vi "SetBuildVersionCaller.vi"(11 "Command line arguments \nfor the VI":string[](array[string])) -> (2 "Output or error information to include in \nthe CLI for LabVIEW console or log file.":string, 3 "CLI for LabVIEW exit code that the VI returns":i32)   [LabVIEW 2020]
doc: "Calls SetBuildVersion.vi to set the version of the build specification."
uses:
  <vilib>/AppBuilder/AB_API_Simple/Build Specification Version.ctl
  <vilib>/AppBuilder/AB_API_Simple/NI_App_Builder_API.lvlib
  <vilib>/AdvancedString/1D String Array to Delimited String (string).vi
  <vilib>/AdvancedString/Delimited String to 1D String Array (string).vi
panel:
  out "error out":errorcluster
  in  "error in (no error)":errorcluster
  out "Set Version":T1
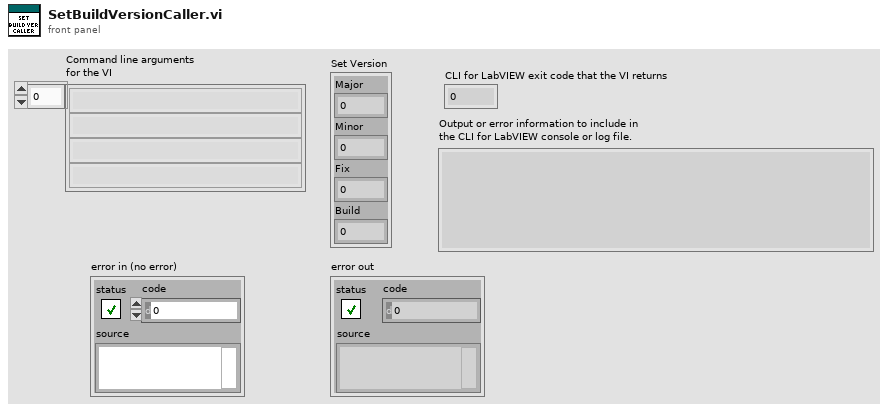
[diagram p1: front panel]
types:
  T1 = typedef "NI_App_Builder_API.lvlib/Build Specification Version.ctl" = cluster{"Major":u16, "Minor":u16, "Fix":u16, "Build":u16}
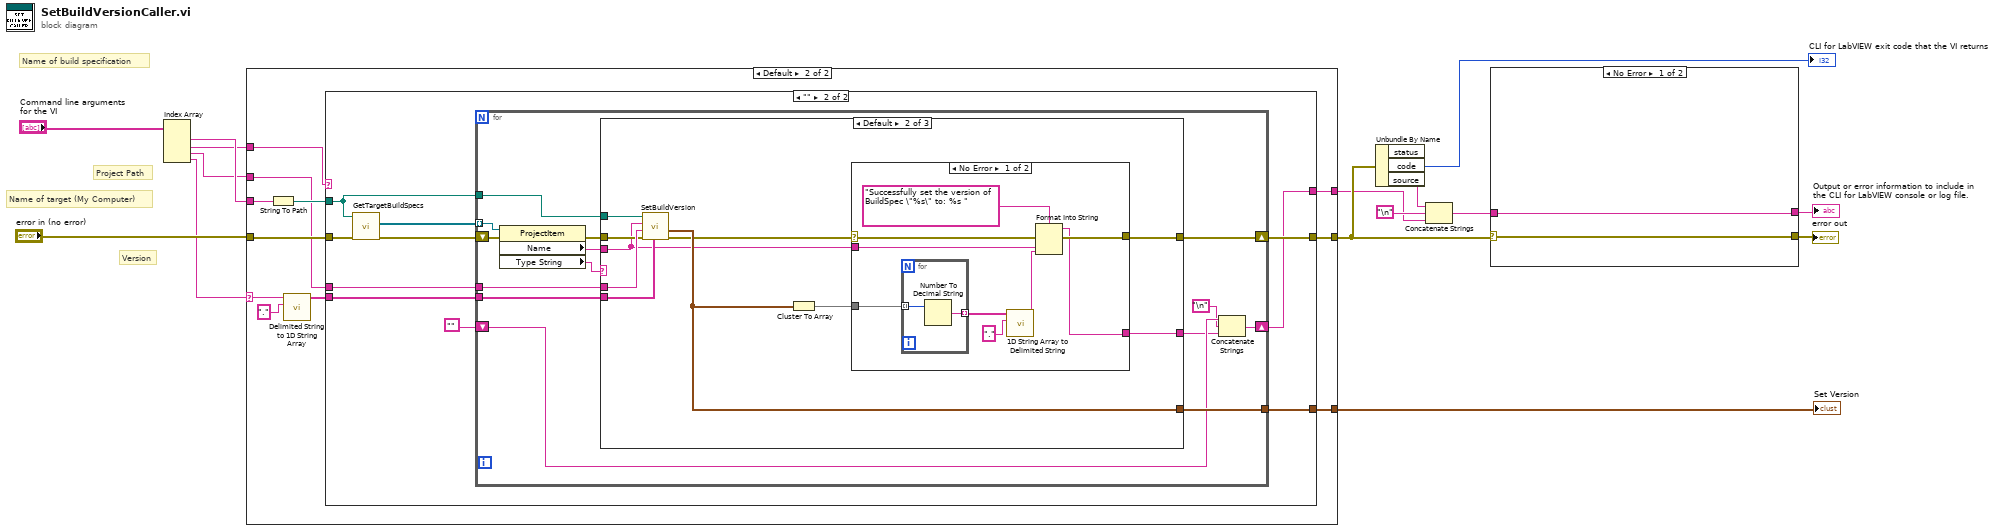
[diagram p0: block diagram]
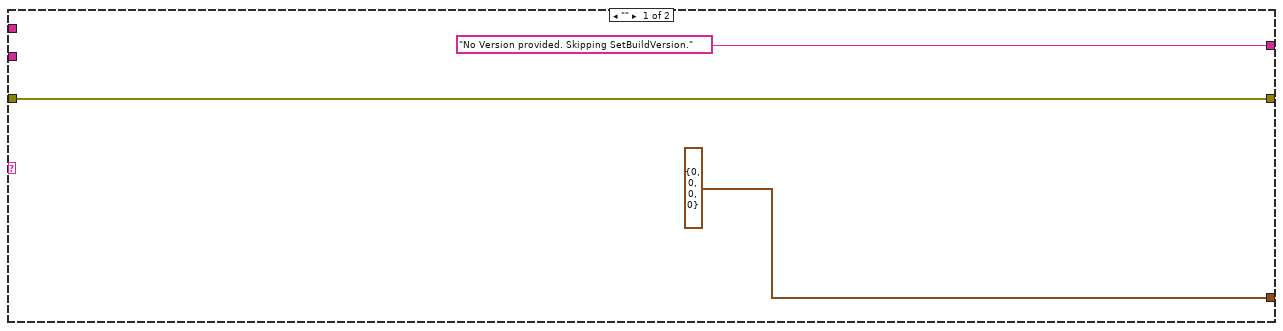
[diagram p3: hidden frame]
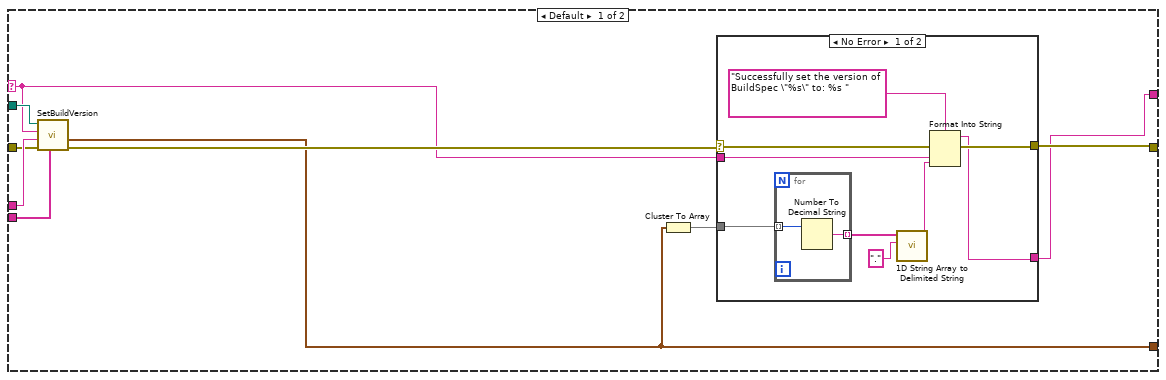
[diagram p4: hidden frame]
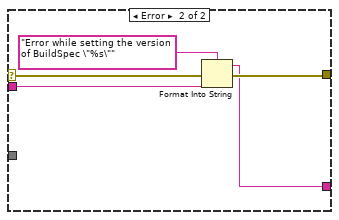
[diagram p5: hidden frame]
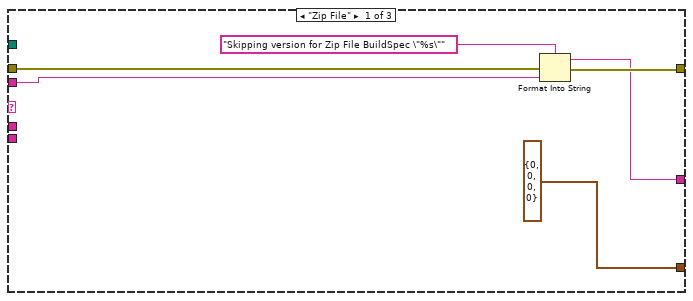
[diagram p6: hidden frame]
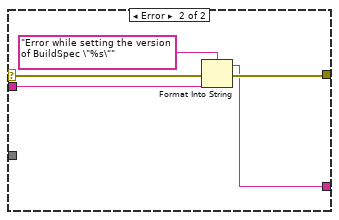
[diagram p7: hidden frame]
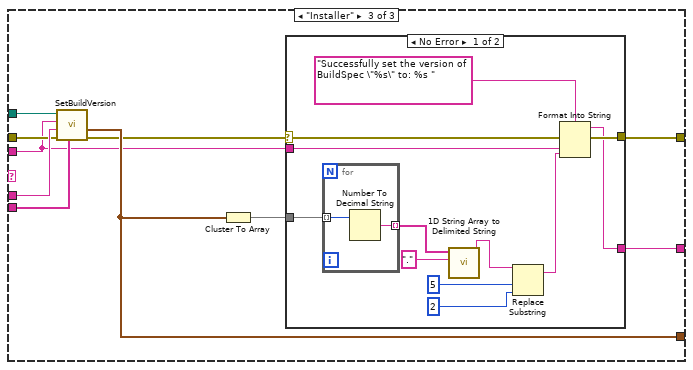
[diagram p8: hidden frame]
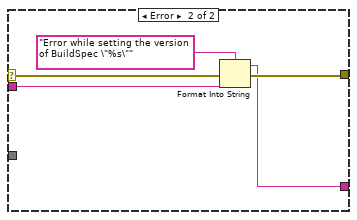
[diagram p9: hidden frame]
diagram:
  # "Project Path"
  # "Version"
  # "Name of target (My Computer)"
  # "Name of build specification"
  n1 = Index Array(array="Command line arguments \nfor the VI") -> (element #1=w14:string, element #2=w11:string, element #3=w12:string, element #4=w10:string)  [unwired: 4 in]
  n2 = case shown="Default" w10 {
    selector: w10 -> [_ w26]
    tunnel: [T1 {"Major"=0, "Minor"=0, "Fix"=0, "Build"=0} ("Set Version") w22] -> w8
    tunnel: ["No Version provided. Skipping SetBuildVersion." ("source") w19] -> w2
    tunnel: [w18 w23] -> w6
    tunnel: w14 -> [_ w28]
    tunnel: "error in (no error)" -> [w18 w24]
    tunnel: w12 -> [_ w21]
    tunnel: w11 -> [_ w27]
    frame "" {
    }
    frame Default {
      n3 = String To Path(string=w28) -> (path=w25:path)
      n4 = call-poly <vilib>:"Delimited String to 1D String Array.vi"("delimiter"=".", "delimited string"=w26) -> ("string array"=w20:string[])  [unwired: 9 in]
      n5 = case shown="\"\"" w27 {
        selector: w27 -> [w33 _]
        tunnel: w25 -> [w36 w58]
        tunnel: w24 -> [w37 w64]
        tunnel: [w34 w62] -> w23
        tunnel: [w32 w61] -> w22
        tunnel: w21 -> [w39 w60]
        tunnel: w20 -> [w38 w59]
        tunnel: [w30 w57] -> w19
        frame Default {
          n6 = call "SetBuildVersion.vi"("Version (delimited)"=w38, "error in (no error)"=w37, "Target Name"=w39, "Name of build specification"=w33, "Path to project"=w36) -> ("error out"=w35:errorcluster, "Set Version"=w32:T1)  [unwired: 5 in]
          n7 = Cluster To Array(cluster=w32) -> (array=w31:u16[])
          n8 = case shown="No Error" w35 {
            selector: w35 -> [w47 w54]
            tunnel: [w46 w55] -> w34
            tunnel: w31 -> [w43 _]
            tunnel: w33 -> [w40 w52]
            tunnel: [w41 w51] -> w30
            frame No Error {
              n9 = for {
                tunnel: w43 -> [w50] mode=indexing
                tunnel: [w49] -> w45 mode=indexing
                n10 = Number To Decimal String(number=w50) -> (decimal integer string=w49:string)  [unwired: 1 in]
              }
              n11 = call-poly <vilib>:"1D String Array to Delimited String.vi"("delimiter"=".", "string array"=w45) -> ("delimited string"=w42:string)  [unwired: 9 in]
              n12 = Format Into String(format string="Successfully set the version of BuildSpec \"%s\" to: %s " ("Text to Write"), error in=w47, w40, w42) -> (resulting string=w41:string, error out=w46:errorcluster)  [unwired: 1 in]
            }
            frame Error {
              n13 = Format Into String(format string="Error while setting the version of BuildSpec \"%s\"" ("Text to Write"), error in=w54, w52) -> (resulting string=w51:string, error out=w55:errorcluster)  [unwired: 1 in]
            }
          }
        }
        frame "" {
          n14 = call <vilib>:"GetTargetBuildSpecs.vi"("error in (no error)"=w64, "Path to project"=w58) -> ("error out"=w63:errorcluster, "buildspec refs"=w65:refnum<vi>[])  [unwired: 2 in, 6 out]
          n15 = for {
            tunnel: w65 -> [w79] mode=indexing
            shift-right: [w68] -> w62
            shift-left: w63 -> [w75]
            tunnel: [w72] -> w61
            tunnel: w60 -> [w78]
            tunnel: w59 -> [w77]
            tunnel: w58 -> [w76]
            shift-right: [w70] -> w57
            shift-left: "" ("Empty String Constant") -> [w71]
            n16 = property on="Property Node" class="ProjectItem"(reference=w79, error in=w75) -> (error out=w74:errorcluster, "Name"=w66:string, "Type String"=w73:string)  [unwired: 1 out]
            n17 = case shown="Default" w73 {
              tunnel: [w83 w88 w114] -> w68
              tunnel: [T1 {"Major"=0, "Minor"=0, "Fix"=0, "Build"=0} ("Set Version") w91 w117] -> w72
              tunnel: w78 -> [_ w95 w121]
              tunnel: w77 -> [_ w94 w120]
              tunnel: w66 -> [w80 w86 w112]
              tunnel: w76 -> [_ w93 w119]
              tunnel: w74 -> [w84 w92 w118]
              tunnel: [w82 w87 w113] -> w67
              frame "Zip File" {
                n18 = Format Into String(format string="Skipping version for Zip File BuildSpec \"%s\"", error in=w84, w80) -> (resulting string=w82:string, error out=w83:errorcluster)  [unwired: 1 in]
              }
              frame Default {
                n19 = call "SetBuildVersion.vi"("Version (delimited)"=w94, "error in (no error)"=w92, "Target Name"=w95, "Name of build specification"=w86, "Path to project"=w93) -> ("error out"=w89:errorcluster, "Set Version"=w91:T1)  [unwired: 5 in]
                n20 = Cluster To Array(cluster=w91) -> (array=w90:u16[])
                n21 = case shown="No Error" w89 {
                  selector: w89 -> [w103 w110]
                  tunnel: [w102 w111] -> w88
                  tunnel: w90 -> [w99 _]
                  tunnel: w86 -> [w96 w108]
                  tunnel: [w97 w107] -> w87
                  frame No Error {
                    n22 = for {
                      tunnel: w99 -> [w106] mode=indexing
                      tunnel: [w105] -> w101 mode=indexing
                      n23 = Number To Decimal String(number=w106) -> (decimal integer string=w105:string)  [unwired: 1 in]
                    }
                    n24 = call-poly <vilib>:"1D String Array to Delimited String.vi"("delimiter"=".", "string array"=w101) -> ("delimited string"=w98:string)  [unwired: 9 in]
                    n25 = Format Into String(format string="Successfully set the version of BuildSpec \"%s\" to: %s " ("Text to Write"), error in=w103, w96, w98) -> (resulting string=w97:string, error out=w102:errorcluster)  [unwired: 1 in]
                  }
                  frame Error {
                    n26 = Format Into String(format string="Error while setting the version of BuildSpec \"%s\"" ("Text to Write"), error in=w110, w108) -> (resulting string=w107:string, error out=w111:errorcluster)  [unwired: 1 in]
                  }
                }
              }
              frame "Installer" {
                n27 = call "SetBuildVersion.vi"("Version (delimited)"=w120, "error in (no error)"=w118, "Target Name"=w121, "Name of build specification"=w112, "Path to project"=w119) -> ("error out"=w115:errorcluster, "Set Version"=w117:T1)  [unwired: 5 in]
                n28 = Cluster To Array(cluster=w117) -> (array=w116:u16[])
                n29 = case shown="No Error" w115 {
                  selector: w115 -> [w132 w139]
                  tunnel: [w131 w140] -> w114
                  tunnel: w116 -> [w128 _]
                  tunnel: w112 -> [w122 w137]
                  tunnel: [w127 w136] -> w113
                  frame No Error {
                    n30 = for {
                      tunnel: w128 -> [w135] mode=indexing
                      tunnel: [w134] -> w130 mode=indexing
                      n31 = Number To Decimal String(number=w135) -> (decimal integer string=w134:string)  [unwired: 1 in]
                    }
                    n32 = call-poly <vilib>:"1D String Array to Delimited String.vi"("delimiter"=".", "string array"=w130) -> ("delimited string"=w126:string)  [unwired: 9 in]
                    n33 = Replace Substring(2:2 ("length (len. of substring)"), 3:5 ("offset (0)"), 5:w126) -> (1:w124:string)  [unwired: 1 in, 1 out]
                    n34 = Format Into String(format string="Successfully set the version of BuildSpec \"%s\" to: %s " ("Text to Write"), error in=w132, w122, w124) -> (resulting string=w127:string, error out=w131:errorcluster)  [unwired: 1 in]
                  }
                  frame Error {
                    n35 = Format Into String(format string="Error while setting the version of BuildSpec \"%s\"" ("Text to Write"), error in=w139, w137) -> (resulting string=w136:string, error out=w140:errorcluster)  [unwired: 1 in]
                  }
                }
              }
            }
            n36 = Concatenate Strings(w71, "\n" ("Line Feed Constant"), w67) -> (w70:string)
          }
        }
      }
    }
  }
  "Set Version" <- w8
  n37 = Unbundle By Name(w6) -> ("code"=→"CLI for LabVIEW exit code that the VI returns":i32, "source"=w4:string)  [unwired: 1 out]
  n38 = Concatenate Strings(w4, "\n" ("Line Feed Constant"), w2) -> (w1:string)
  n39 = case shown="No Error" w6 {
    selector: w6 -> [w142 w144]
    tunnel: [w142 w144] -> w9
    tunnel: [w141 w143] -> w7
    tunnel: w1 -> [w141 w143]
    frame No Error {
    }
    frame Error {
    }
  }
  "error out" <- w9
  "Output or error information to include in \nthe CLI for LabVIEW console or log file." <- w7
